vi "Read Event_Source.vi"(8 "error in (no error)":errorcluster, 11 "Event_Bus in":refnum<class "Event_Bus.lvclass">) -> (0 "error out":errorcluster, 2 "Event_Source.lvclass":refnum<class "Event_Source.lvclass">, 3 "Event_Bus out":refnum<class "Event_Bus.lvclass">)   [LabVIEW 2021, in "Event_Bus.lvclass"]
uses:
  Event_Bus.lvclass
  Support/Event Source/Event_Source.lvclass
  Event_Bus.lvclass/Event_Bus.ctl
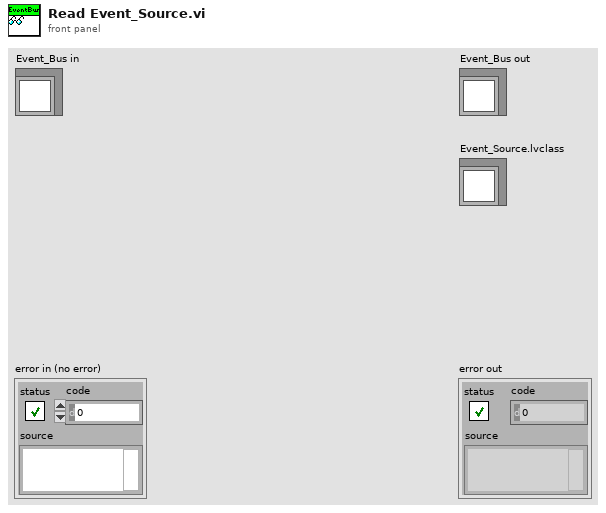
[diagram p1: front panel]
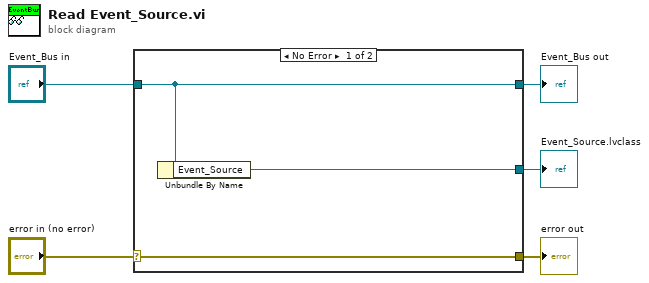
[diagram p0: block diagram]
diagram:
  n1 = case shown="No Error" "error in (no error)" {
    selector: "error in (no error)" -> [w8 w9]
    tunnel: [w8 w9] -> w4
    tunnel: [w7 w10] -> w2
    tunnel: "Event_Bus in" -> [w7 w10]
    tunnel: [w6 _] -> w1
    frame No Error {
      n2 = Unbundle By Name(w7) -> ("Event_Source"=w6:refnum<class "Event_Source.lvclass">)
    }
    frame Error {
    }
  }
  "error out" <- w4
  "Event_Bus out" <- w2
  "Event_Source.lvclass" <- w1
